vi "Channel_Equal.vi"(0 "cellid":dbl, 2 "error in (no error)":errorcluster caption="错误输入（无错误）", 6 "UL_subframe_num":dbl, 7 "antnum":dbl, 8 "rbstart":dbl, 9 "prb_num":dbl, 10 "freqdata":cdb[][](array[numeric]), 11 "appended path":path) -> (1 "error IO":errorcluster, 3 "equfredata":cdb[][](array[numeric]), 4 "slot1_lschannel":cdb[](array[numeric]), 5 "slot0_lschannel":cdb[](array[numeric]))   [LabVIEW 2015]
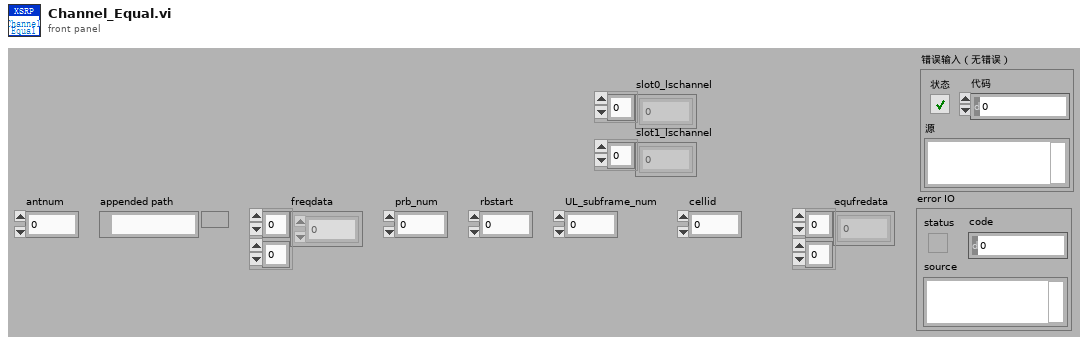
[diagram p1: front panel]
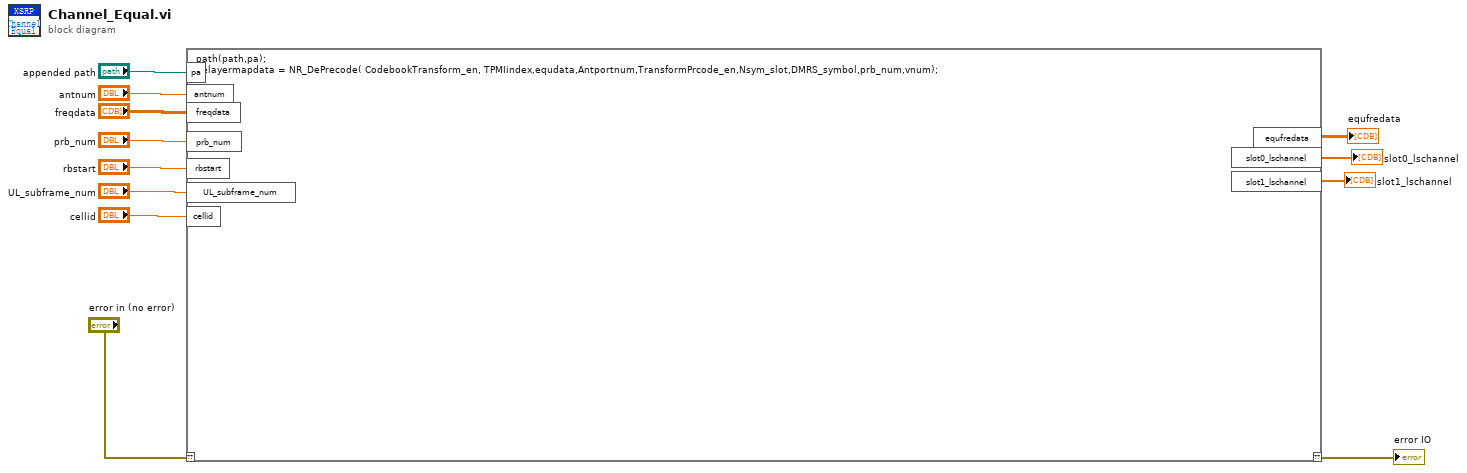
[diagram p0: block diagram]
diagram:
  n1 = script code="path(path,pa);\ndelayermapdata = NR_DePrecode( CodebookTransform_en, TPMIindex,equdata,Antportnum,TransformPrcode_en,Nsym_slot,DMRS_symbol,prb_num,vnum);"("??"="error in (no error)", "pa"="appended path", "antnum"="antnum", "freqdata"="freqdata", "prb_num"="prb_num", "rbstart"="rbstart", "UL_subframe_num"="UL_subframe_num", "cellid"="cellid") -> ("??"=→"error IO":errorcluster, "equfredata"=→"equfredata":cdb[][], "slot0_lschannel"=→"slot0_lschannel":cdb[], "slot1_lschannel"=→"slot1_lschannel":cdb[])
